vi "LED_Globals.vi"() -> ()   [LabVIEW 2019]
panel:
  in  "LED_CANifier":string="LED_CANifier"
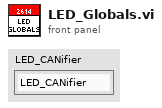
[diagram p1: front panel]
diagram:
